vi "Create Oneof Case Structure.vi"(8 "error in (no error)":errorcluster, 10 "Oneof Container Name":string, 11 "VI in":refnum<vi>) -> (0 "error out":errorcluster, 2 "CaseStructure out":refnum<vi>, 3 "VI out":refnum<vi>)   [LabVIEW 2019, in "gRPC Template Creation Utility.lvlib"]
uses:
  gRPC Template Creation Utility.lvlib
panel:
  # "Creates only a single frame with default case\nfor selected index of the oneof."
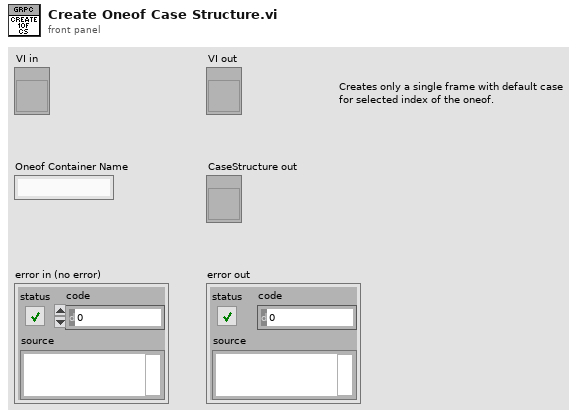
[diagram p1: front panel]
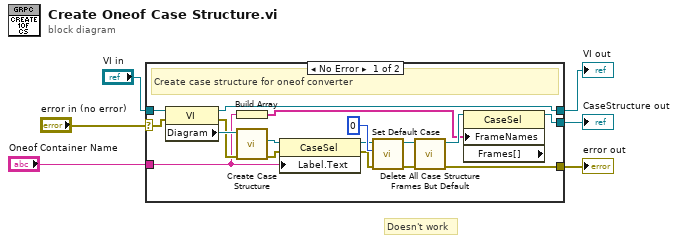
[diagram p0: block diagram]
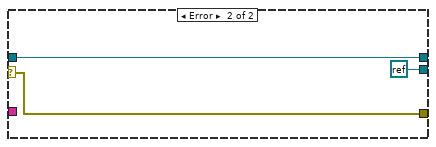
[diagram p2: hidden frame]
diagram:
  # "Doesn't work"
  n1 = case shown="No Error" "error in (no error)" {
    selector: "error in (no error)" -> [w22 w25]
    tunnel: "Oneof Container Name" -> [w7 _]
    tunnel: "VI in" -> [w23 w26]
    tunnel: [w21 w25] -> w3
    tunnel: [w11 w26] -> w2
    tunnel: [w9 refnum<k0> refnum] -> w1
    frame No Error {
      # "Create case structure for oneof converter"
      n2 = property class="VI"(reference=w23, error in=w22) -> (reference out=w11:refnum<vi>, error out=w19:errorcluster, "Diagram"=w20:refnum<vi>)
      n3 = Build Array(w7) -> (w8:string[])
      n4 = call "Create Case Structure.vi"("error in (no error)"=w19, "Block Diagram in"=w20) -> ("error out"=w17:errorcluster, "Case Structure out"=w18:refnum<vi>)  [unwired: 7 in, 1 out]
      n5 = property class="CaseSel"(reference=w18, error in=w17, "Label.Text"=w7) -> (reference out=w14:refnum<vi>, error out=w13:errorcluster)
      n6 = call "Set Default Case.vi"("error in (no error)"=w13, "Case Index"=0, "Case Structure in"=w14) -> ("error out"=w12:errorcluster, "Case Structure out"=w15:refnum<vi>)  [unwired: 7 in]
      n7 = call "Delete All Case Structure Frames But Default.vi"("error in (no error)"=w12, "CaseStructure in"=w15) -> ("error out"=w21:errorcluster, "CaseStructure out"=w10:refnum<vi>)  [unwired: 8 in]
      n8 = property class="CaseSel" props=["FrameNames", "Frames[]"](reference=w10, "FrameNames"=w8) -> (reference out=w9:refnum<vi>)  [unwired: 1 in, 2 out]
    }
    frame Error {
    }
  }
  "error out" <- w3
  "VI out" <- w2
  "CaseStructure out" <- w1
